vi "Transmit.vi"(4 "Len":u32, 6 "pSend":u8[](array[numeric]), 8 "error in (no error)":errorcluster caption="错误输入（无错误）", 9 "CANInd":u32, 10 "DeviceInd":u32, 11 "type":u16(ring)=2 items=["USB-CAN"=2, "USB-CAN2.0"=3]) -> (0 "error out":errorcluster caption="错误输出", 3 "Success":u32)   [LabVIEW 2011]
uses:
  data/ControlCAN.dll
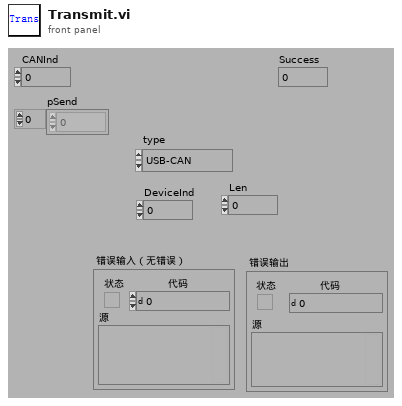
[diagram p1: front panel]
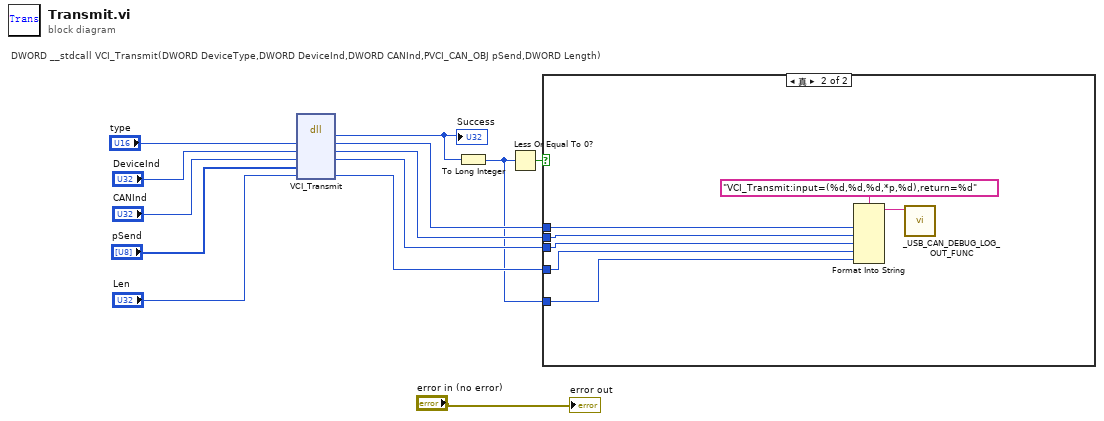
[diagram p0: block diagram]
diagram:
  # "DWORD __stdcall VCI_Transmit(DWORD DeviceType,DWORD DeviceInd,DWORD CANInd,PVCI_CAN_OBJ pSend,DWORD Length)"
  n1 = dll-call lib="PTH1Mabs ZHost_E工作TnewcodeUSB CAN Tool1.97dataControlCAN.dll" fn="VCI_Transmit"("DeviceType"="type", "DeviceInd"="DeviceInd", "CANInd"="CANInd", "pSend"="pSend", "Len"="Len") -> ("返回类型"=w7:u32, "DeviceType"=w5:u32, "DeviceInd"=w4:u32, "CANInd"=w3:u32, "Len"=w2:u32)  [unwired: 4 in, 2 out]
  "Success" <- w7
  n2 = To Long Integer(number=w7) -> (32bit integer=w1:i32)
  n3 = Less Or Equal To 0?(x=w1) -> (x <= 0?=w6:bool)
  n4 = case shown="真" w6 {
    tunnel: w5 -> [_ w18]
    tunnel: w4 -> [_ w17]
    tunnel: w3 -> [_ w16]
    tunnel: w2 -> [_ w15]
    tunnel: w1 -> [_ w14]
    frame False {
    }
    frame True {
      n5 = Format Into String(format string="VCI_Transmit:input=(%d,%d,%d,*p,%d),return=%d", w18, w17, w16, w15, w14) -> (resulting string=w19:string)  [unwired: 2 in, 1 out]
      n6 = call "_USB_CAN_DEBUG_LOG_OUT_FUNC.vi"("Info"=w19) -> ()  [unwired: 11 in]
    }
  }
  "error out" <- "error in (no error)"
